vi "prep.vi"(8 "error in (no error)":errorcluster, 9 "Coordinate System":enum16{"Cartesian", "Cylindrical", "Spherical"}(ring), 10 "Plot processed data In":T1 caption="Data In", 11 "Base Datatype in":refnum<class "Base Datatype.lvclass">) -> (0 "error out":errorcluster, 2 "Plot processed Data Out":T1 caption="Data Out", 3 "Base Datatype out":refnum<class "Base Datatype.lvclass">)   [LabVIEW 2017, in "Base Datatype.lvclass"]
uses:
  <vilib>/Native 3D Graph/classes/Base Datatype.lvclass
  <vilib>/Native 3D Graph/xcontrol/Processed Data.ctl
  <vilib>/Native 3D Graph/typedefs/plot_rep_array.ctl
  <vilib>/Native 3D Graph/typedefs/plot_rep.ctl
  <vilib>/Native 3D Graph/typedefs/range_cluster.ctl
  <vilib>/Native 3D Graph/typedefs/min_max.ctl
  <vilib>/Native 3D Graph/typedefs/plot_rep_mesh_data.ctl
  <vilib>/Native 3D Graph/xcontrol/3DPC_SurfacePlot.xctl
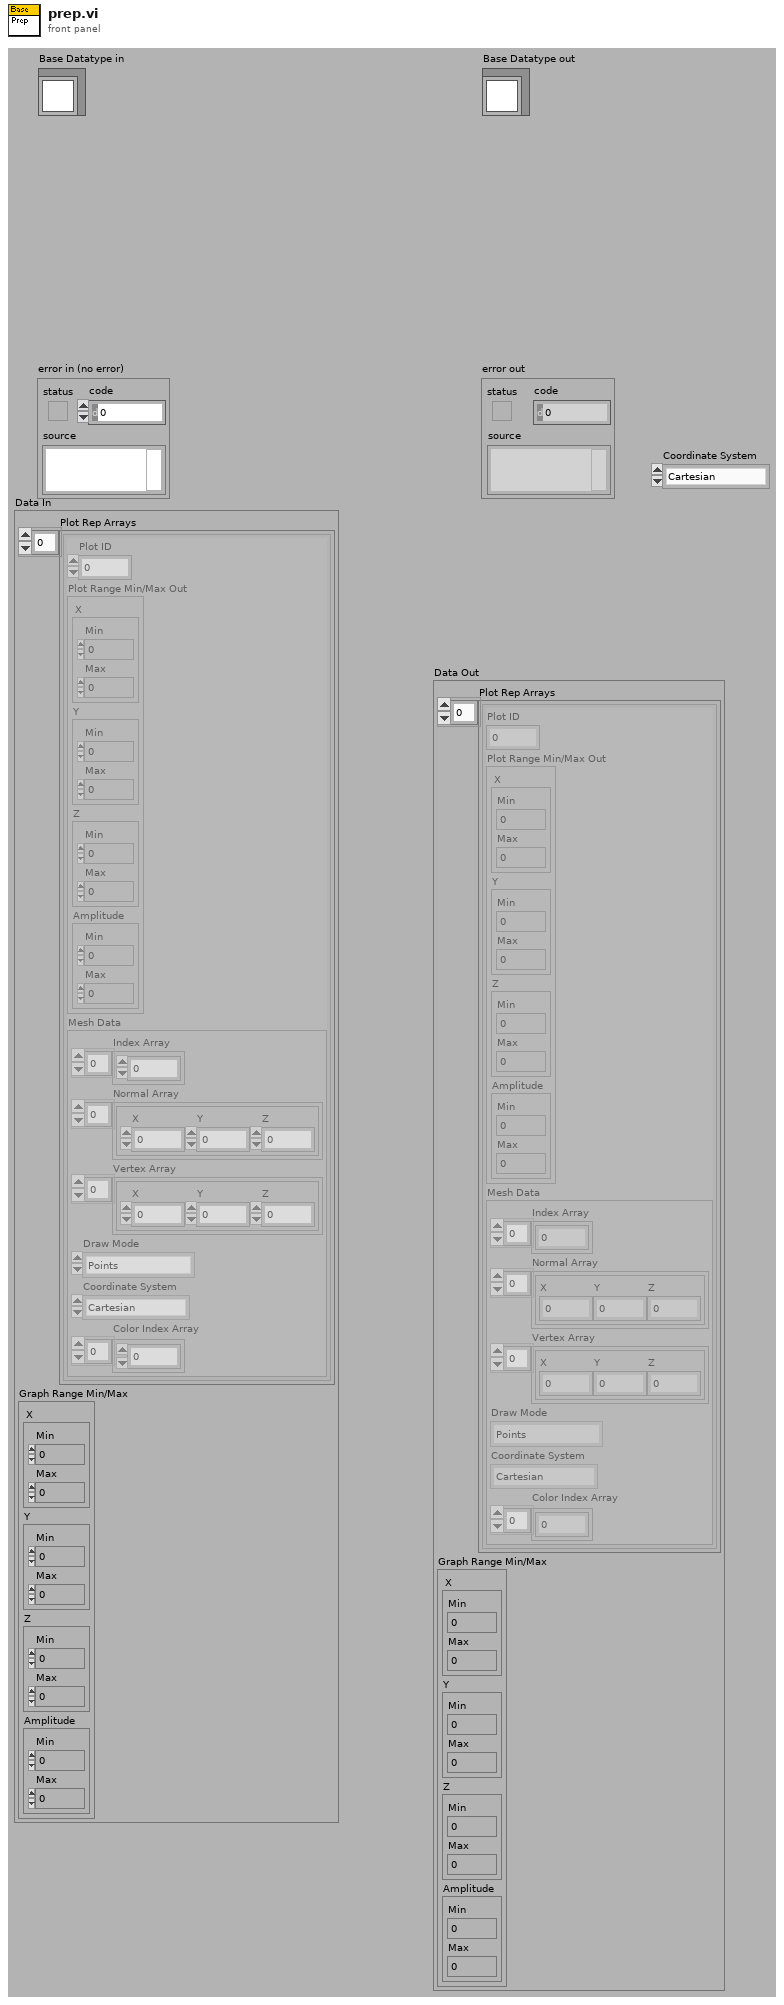
[diagram p1: front panel]
types:
  T1 = typedef "Processed Data.ctl" = cluster{"Plot Rep Arrays":T2, "Graph Range Min/Max":T4}
  T2 = typedef "3DPC_SurfacePlot.xctl/plot_rep_array.ctl" = T3[]
  T3 = typedef "3DPC_SurfacePlot.xctl/plot_rep.ctl" = cluster{"Plot ID":i32, "Plot Range Min/Max Out":T4, "Mesh Data":T6}
  T4 = typedef "3DPC_SurfacePlot.xctl/range_cluster.ctl" = cluster{"X":T5, "Y":T5, "Z":T5, "Amplitude":T5}
  T5 = typedef "3DPC_SurfacePlot.xctl/min_max.ctl" = cluster{"Min":sgl, "Max":sgl}
  T6 = typedef "3DPC_SurfacePlot.xctl/plot_rep_mesh_data.ctl" = cluster{"Index Array":u32[], "Normal Array":cluster{"X":sgl, "Y":sgl, "Z":sgl}[], "Vertex Array":cluster{"X":sgl, "Y":sgl, "Z":sgl}[], "Draw Mode":enum16{"Points", "Lines", "Line Strip", "Line Loop", "Triangles", "Triangle Strip", "Triangle Fan", "Quads", "Quad Strip", "Polygon"}, "Coordinate System":enum16{"Cartesian", "Cylindrical", "Spherical"}, "Color Index Array":i32[]}
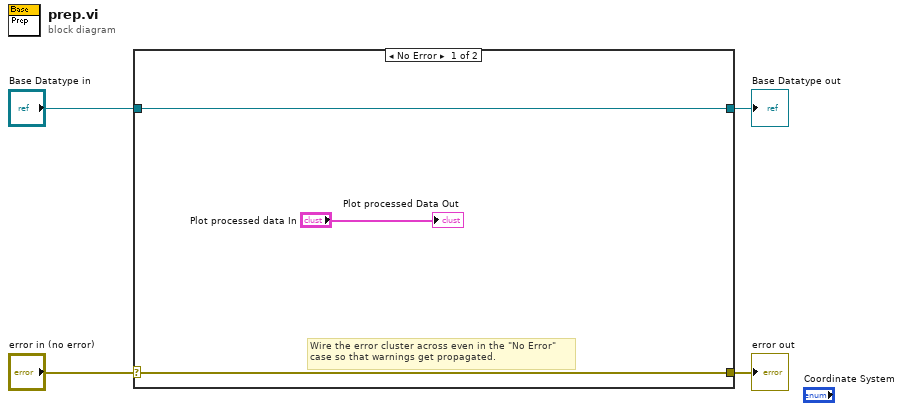
[diagram p0: block diagram]
diagram:
  n1 = case shown="No Error" "error in (no error)" {
    selector: "error in (no error)" -> [w6 w9]
    tunnel: [w6 w9] -> w3
    tunnel: [w7 w8] -> w1
    tunnel: "Base Datatype in" -> [w7 w8]
    frame No Error {
      # "Wire the error cluster across even in the \"No Error\"\ncase so that warnings get propagated."
      "Plot processed Data Out" <- "Plot processed data In"
    }
    frame Error {
    }
  }
  "error out" <- w3
  "Base Datatype out" <- w1
